vi "Host_RUNPARAMETERS.vi"() -> ()   [LabVIEW 2018]
uses:
  Master/TypeDef_RunParameters.ctl
panel:
  in  "Service Parameters":T1 {"Target (I16)" min=0 max=5 step=1}
  in  "Full Run Parameters":T1 {"Target (I16)" min=0 max=5 step=1}
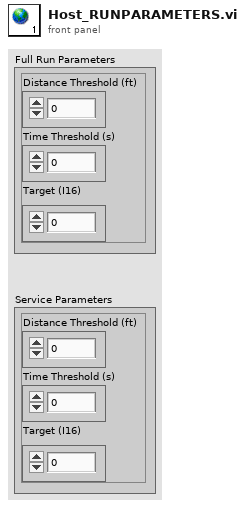
[diagram p1: front panel]
types:
  T1 = typedef "TypeDef_RunParameters.ctl" = cluster{"Distance Threshold (ft)":dbl, "Time Threshold (s)":dbl, "Target (I16)":i16}
diagram:
